vi "Write Wavelength.vi"(8 "error in (no error)":errorcluster, 10 "Wavelength (nm)":dbl, 11 "EXFO in":refnum<class "EXFO.lvclass">) -> (0 "error out":errorcluster, 3 "EXFO out":refnum<class "EXFO.lvclass">)   [LabVIEW 2018, in "EXFO.lvlib" / "EXFO.lvclass"]
doc: "This is an override VI, call parent method before or after child method overrites it. Write the target wavelength to the EXFO. For Luminar the wavelength should be 1550 nm. If there is a tolerance, make sure it does not exceed +-5 nm or we risk violating ITAR\n\nAuthor: Ron Dexter\nCompany: Luminar\nModified: 5/20/2018"
uses:
  EXFO.lvclass
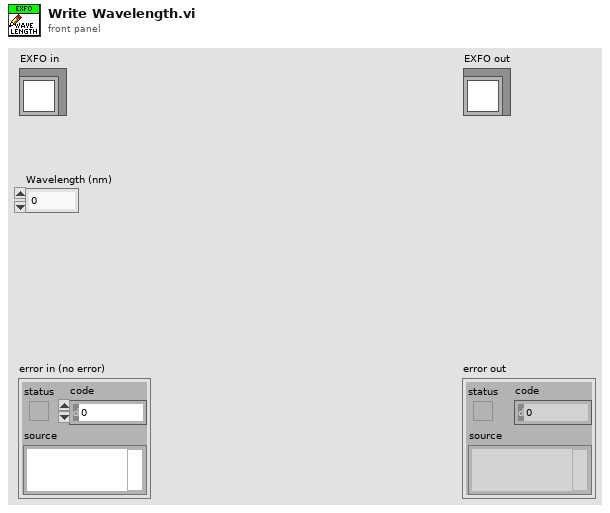
[diagram p1: front panel]
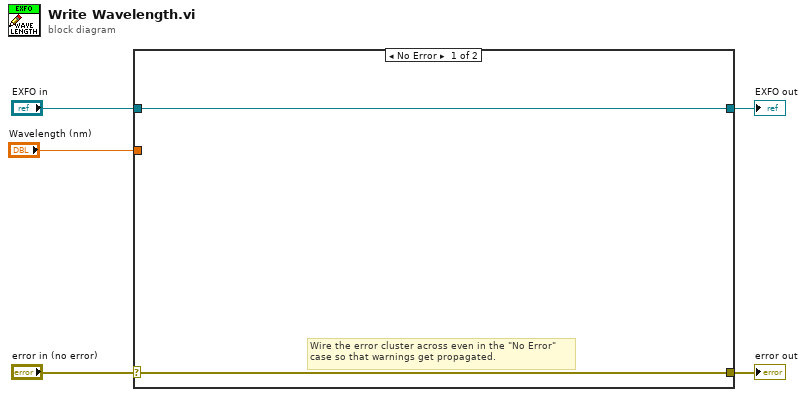
[diagram p0: block diagram]
diagram:
  n1 = case shown="No Error" "error in (no error)" {
    selector: "error in (no error)" -> [w7 w9]
    tunnel: [w7 w9] -> w4
    tunnel: [w6 w8] -> w2
    tunnel: "EXFO in" -> [w6 w8]
    tunnel: "Wavelength (nm)" -> [_ _]
    frame No Error {
      # "Wire the error cluster across even in the \"No Error\"\ncase so that warnings get propagated."
    }
    frame Error {
    }
  }
  "error out" <- w4
  "EXFO out" <- w2
